vi "roboLV2.vi"() -> ()   [LabVIEW 2013]
uses:
  <vilib>/Instr/_visa.llb/VISA Configure Serial Port (Instr).vi
panel:
  out "Elbow Waveform":dbl(graph)
  out "Elbow":dbl[](array[numeric])
  out "Gripper":bool
  out "Wrist":bool
  out "Elbow":bool
  out "Shoulder":bool
  out "Base":bool
  out "Wrist Waveform":dbl(graph)
  out "Shoulder Waveform":dbl(graph)
  out "String":string
  out "Numeric":dbl
  out "Wrist":dbl[](array[numeric])
  out "Shoulder":dbl[](array[numeric])
  in  "Clear":bool
  in  "?":bool
  out "?":bool
  out "Motor":u32
  in  "VISA resource name":refnum<visa-resource-name>
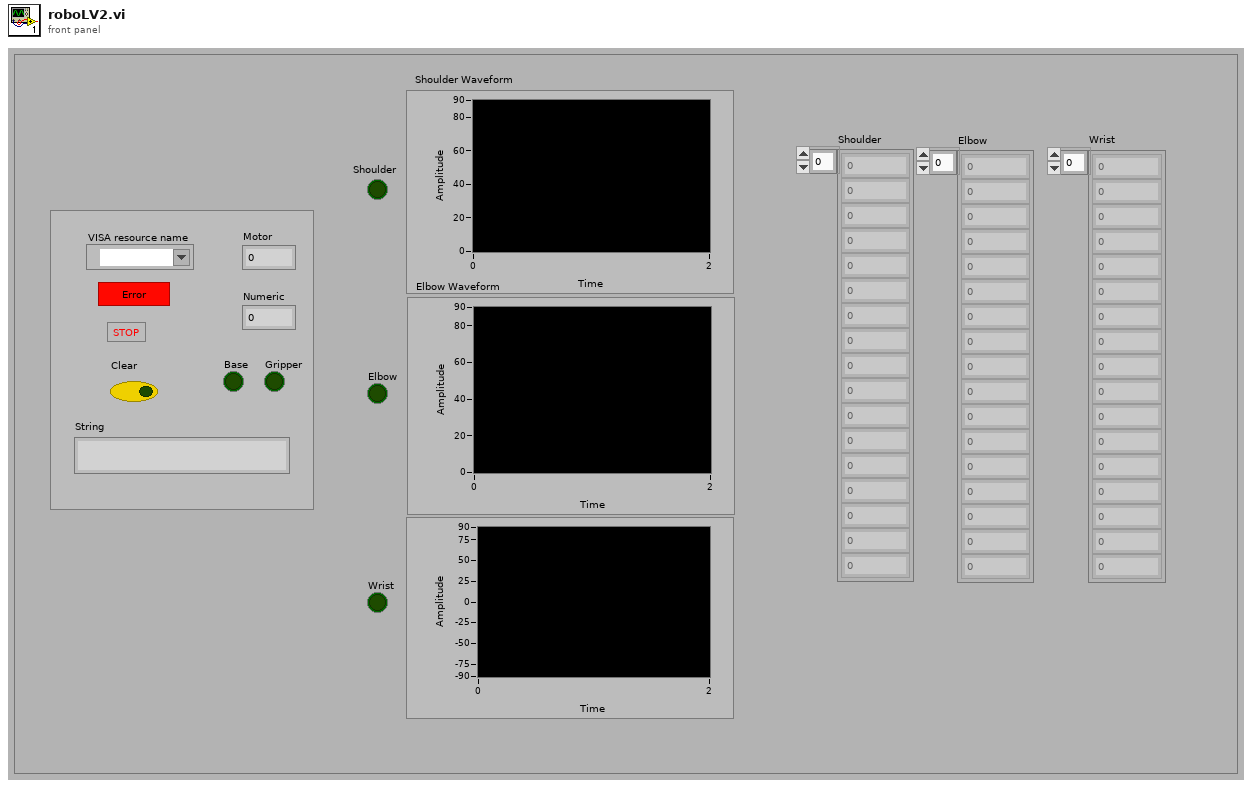
[diagram p1: front panel]
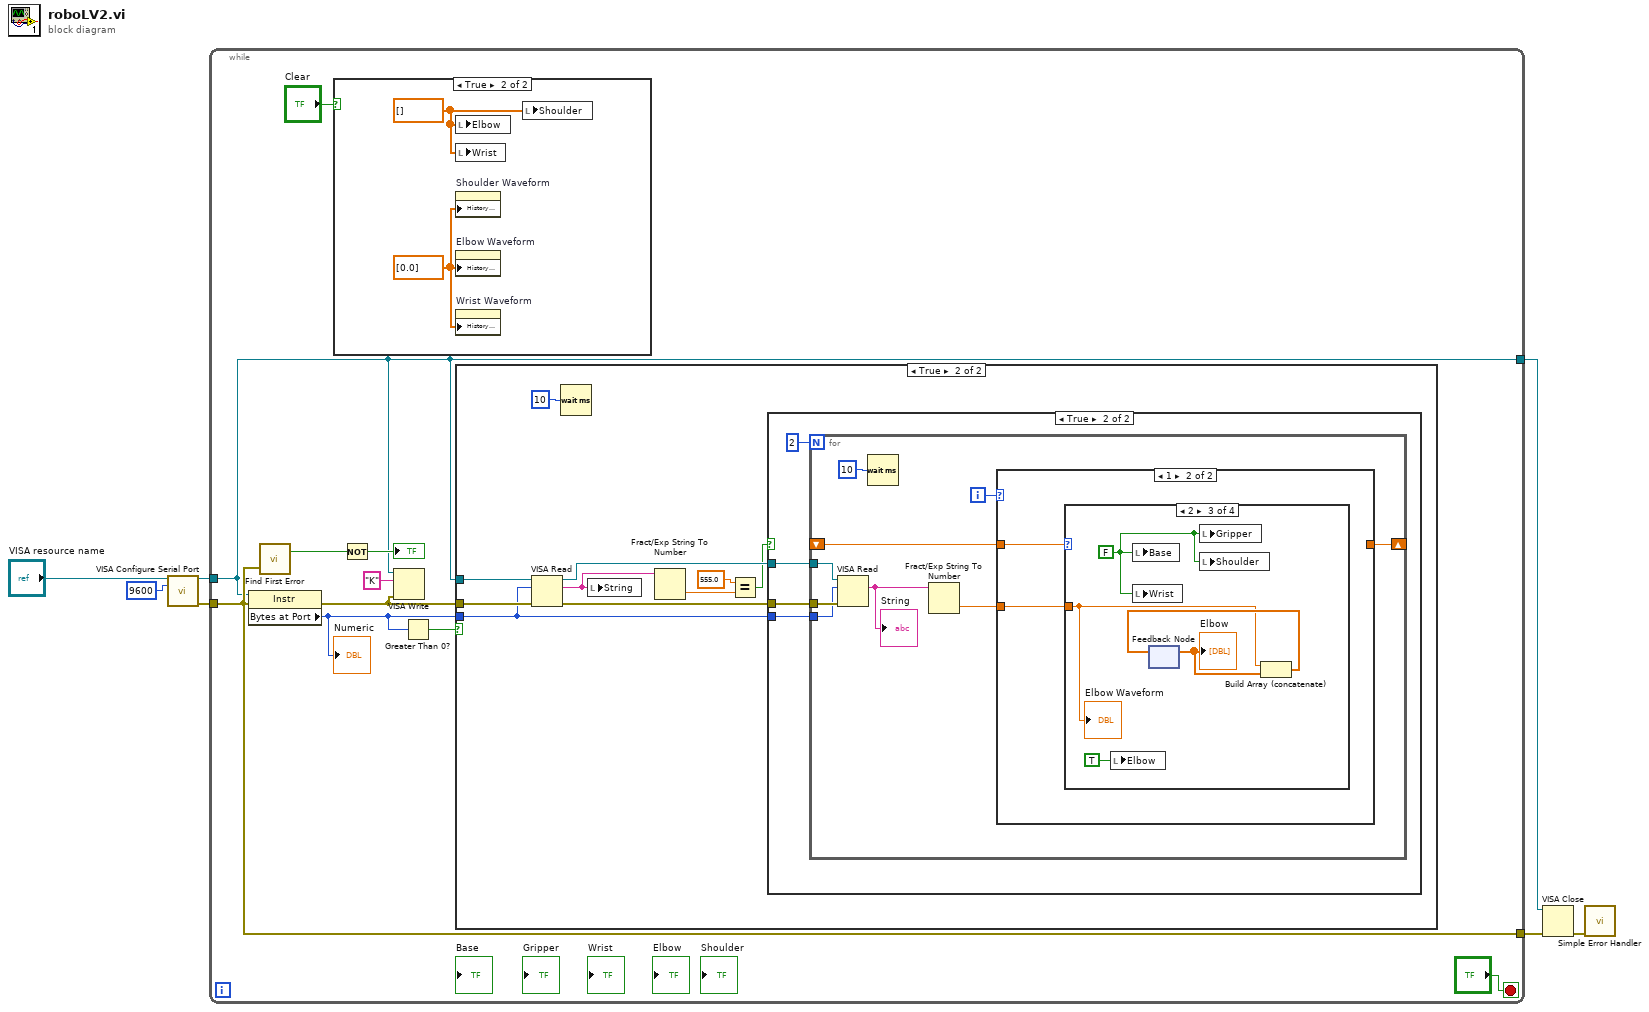
[diagram p0: block diagram]
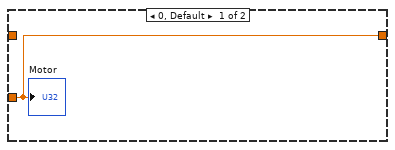
[diagram p4: hidden frame]
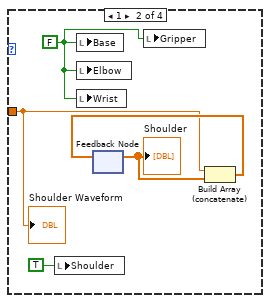
[diagram p6: hidden frame]
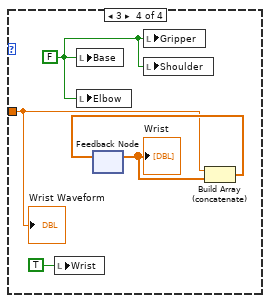
[diagram p7: hidden frame]
diagram:
  n1 = call-poly "VISA Configure Serial Port"("VISA resource name"="VISA resource name", "baud rate (9600)"=u32 9600) -> ("VISA resource name out"=w3:refnum<visa-resource-name>, "error out"=w4:errorcluster)  [unwired: 12 in]
  n2 = while {
    tunnel: w4 -> [w15]
    tunnel: w3 -> [w12]
    tunnel: [w15] -> w2
    tunnel: [w12] -> w1
    stop <- "?" stop-if-true
    n3 = property class="Instr"(reference=w12, error in=w15) -> (error out=w11:errorcluster, "Bytes at Port"=w8:u32)  [unwired: 1 out]
    "Numeric" <- w8
    n4 = call <vilib>:"Find First Error.vi"("error in (no error)"=w15) -> ("error?"=w17:bool)  [unwired: 3 in, 1 out]
    n5 = case shown="True" "Clear" {
      frame False {
      }
      frame True {
        w60 = dbl[] [0.0] ("History Data")
        w59 = dbl[] [] ("History Data")
        n6 = local write "Elbow"(w59) -> ()
        n7 = local write "Wrist"(w59) -> ()
        n8 = property on="Shoulder Waveform" class="WFChart (strict)"("History Data"=w60) -> ()  [unwired: 2 in, 2 out]
        n9 = property on="Elbow Waveform" class="WFChart (strict)"("History Data"=w60) -> ()  [unwired: 2 in, 2 out]
        n10 = property on="Wrist Waveform" class="WFChart (strict)"("History Data"=w60) -> ()  [unwired: 2 in, 2 out]
        n11 = local write "Shoulder"(w59) -> ()
      }
    }
    n12 = Not(x=w17) -> (.not. x?=→"?":bool)
    n13 = VISA Write(VISA resource name=w12, write buffer="K", error in (no error)=w11) -> ()  [unwired: 3 out]
    n14 = Greater Than 0?(x=w8) -> (x > 0?=w10:bool)
    n15 = case shown="True" w10 {
      tunnel: w8 -> [_ w23]
      tunnel: w12 -> [_ w24]
      tunnel: w11 -> [_ w26]
      frame False {
      }
      frame True {
        n16 = VISA Read(VISA resource name=w24, byte count=w23, error in (no error)=w26) -> (VISA resource name out=w25:refnum<visa-resource-name>, read buffer=w21:string, error out=w27:errorcluster)  [unwired: 1 out]
        n17 = Wait (ms)(milliseconds to wait=u32 10) -> ()  [unwired: 1 out]
        n18 = local write "String"(w21) -> ()
        n19 = Fract/Exp String To Number(string=w21) -> (number=w20:dbl)  [unwired: 3 in, 1 out]
        n20 = Equal?(x=555.0, y=w20) -> (x = y?=w22:bool)
        n21 = case shown="True" w22 {
          tunnel: w27 -> [_ w30]
          tunnel: w25 -> [_ w29]
          tunnel: w23 -> [_ w28]
          frame False {
          }
          frame True {
            n22 = for {
              N: 2 -> [_]
              tunnel: w29 -> [w40]
              tunnel: w30 -> [w39]
              tunnel: w28 -> [w38]
              shift-right: [w34] -> _
              shift-left: _ -> [w33]
              i -> [w37]
              n23 = VISA Read(VISA resource name=w40, byte count=w38, error in (no error)=w39) -> (read buffer=w35:string)  [unwired: 3 out]
              "String" <- w35
              n24 = Wait (ms)(milliseconds to wait=u32 10) -> ()  [unwired: 1 out]
              n25 = Fract/Exp String To Number(string=w35) -> (number=w36:dbl)  [unwired: 3 in, 1 out]
              n26 = case shown="1" w37 {
                tunnel: w36 -> [w41 w42]
                tunnel: [w41 _] -> w34
                tunnel: w33 -> [_ w43]
                frame 0, Default {
                  "Motor" <- w41
                }
                frame 1 {
                  n27 = case shown="2" w43 {
                    tunnel: w42 -> [_ w47 w52 w56]
                    frame 0, Default {
                    }
                    frame 1 {
                      w45 = FALSE ("Base")
                      n28 = local write "Shoulder"(TRUE ("Shoulder")) -> ()
                      n29 = local write "Base"(w45) -> ()
                      n30 = local write "Elbow"(w45) -> ()
                      n31 = local write "Wrist"(w45) -> ()
                      n32 = feedback #1() -> (w44:dbl[])  [unwired: 1 in]
                      "Shoulder" <- w44
                      n33 = local write "Gripper"(w45) -> ()
                      n34 = Build Array (concatenate)(w47, w44) -> (w48:dbl[])
                      n35 = feedback-in #1(w48) -> ()
                      "Shoulder Waveform" <- w47
                    }
                    frame 2 {
                      w50 = FALSE ("Base")
                      n36 = local write "Elbow"(TRUE ("Shoulder")) -> ()
                      n37 = local write "Base"(w50) -> ()
                      n38 = local write "Wrist"(w50) -> ()
                      n39 = feedback #2() -> (w49:dbl[])  [unwired: 1 in]
                      "Elbow" <- w49
                      n40 = local write "Gripper"(w50) -> ()
                      n41 = local write "Shoulder"(w50) -> ()
                      n42 = Build Array (concatenate)(w52, w49) -> (w53:dbl[])
                      n43 = feedback-in #2(w53) -> ()
                      "Elbow Waveform" <- w52
                    }
                    frame 3 {
                      w54 = FALSE ("Base")
                      n44 = local write "Wrist"(TRUE ("Shoulder")) -> ()
                      n45 = local write "Base"(w54) -> ()
                      n46 = local write "Elbow"(w54) -> ()
                      n47 = feedback #3() -> (w57:dbl[])  [unwired: 1 in]
                      "Wrist" <- w57
                      n48 = local write "Gripper"(w54) -> ()
                      n49 = local write "Shoulder"(w54) -> ()
                      n50 = Build Array (concatenate)(w56, w57) -> (w58:dbl[])
                      n51 = feedback-in #3(w58) -> ()
                      "Wrist Waveform" <- w56
                    }
                  }
                }
              }
            }
          }
        }
      }
    }
  }
  n52 = VISA Close(VISA resource name=w1, error in (no error)=w2) -> (error out=w5:errorcluster)
  n53 = call <vilib>:"Simple Error Handler.vi"("error in (no error)"=w5) -> ()  [unwired: 4 in, 5 out]
